vi "Inject Tip Strip Text.vi"(4 "Active File Not Changed Tip Strip":string, 6 "Active File Changed Tip Strip":string, 11 "Test Executive Builder Dirty Dot View in":refnum<class "Test Executive Builder Dirty Dot View.lvclass">) -> (3 "Test Executive Builder Dirty Dot View out":refnum<class "Test Executive Builder Dirty Dot View.lvclass">)   [LabVIEW 2017, in "Test Executive Builder Dirty Dot View.lvclass"]
uses:
  <vilib>/gpm_packages/@cs/Test-executive-builder/Source/Dirty Dot View/Test Executive Builder Dirty Dot View/Test Executive Builder Dirty Dot View.lvclass
  <vilib>/gpm_packages/@cs/Test-executive-builder/Source/Dirty Dot View/Test Executive Builder Dirty Dot View/Test Executive Builder Dirty Dot View.lvclass/Test Executive Builder Dirty Dot View.ctl
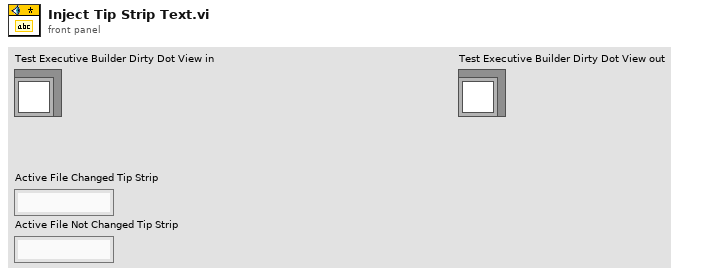
[diagram p1: front panel]
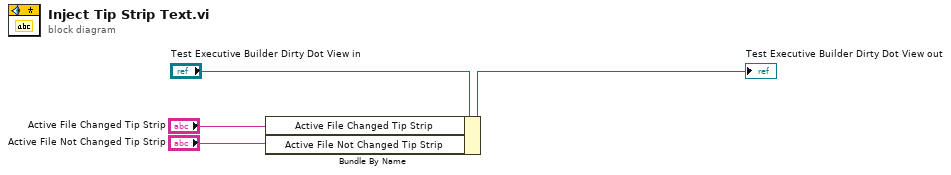
[diagram p0: block diagram]
diagram:
  n1 = Bundle By Name(cluster="Test Executive Builder Dirty Dot View in", "Active File Changed Tip Strip"="Active File Changed Tip Strip", "Active File Not Changed Tip Strip"="Active File Not Changed Tip Strip") -> (→"Test Executive Builder Dirty Dot View out":refnum<class "Test Executive Builder Dirty Dot View.lvclass">)
